vi "KeepScreenTrunOn.vi"(8 "error in (no error)":errorcluster) -> (0 "error out":errorcluster, 3 "PowerHandle":u32)   [LabVIEW 2020, in "Power Requests.lvlib"]
uses:
  Power Requests.lvlib
  Power Availabilty Requests/Type Defs/Power Request Type.ctl
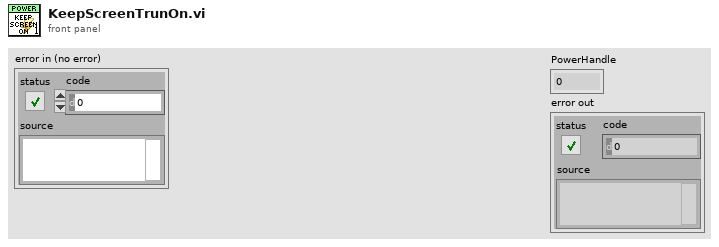
[diagram p1: front panel]
types:
  T1 = typedef "Power Requests.lvlib/Power Request Type.ctl" = enum32{"Power Request Display Required", "Power Request System Required", "Power Request Away Mode Required", "Power Request Execution Required"}
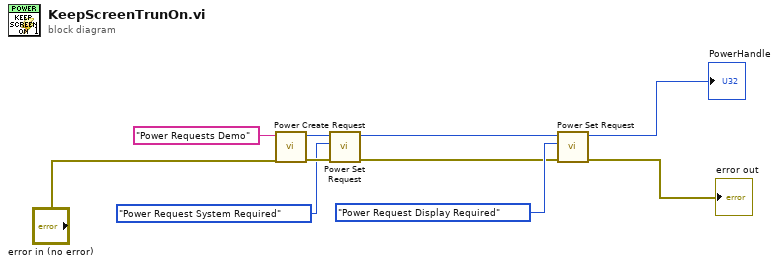
[diagram p0: block diagram]
diagram:
  n1 = call "Power Create Request.vi"("error in (no error)"="error in (no error)", "Simple Reason String"="Power Requests Demo") -> ("error out"=w10:errorcluster, "Handle"=w9:i64)  [unwired: 8 in]
  n2 = call "Power Set Request.vi"("error in (no error)"=w10, "Power Request Type"=Power_Request_Type."Power Request System Required", "Handle in"=w9) -> ("error out"=w5:errorcluster, "Handle out"=w4:u32)  [unwired: 6 in, 1 out]
  n3 = call "Power Set Request.vi"("error in (no error)"=w5, "Power Request Type"=Power_Request_Type."Power Request Display Required", "Handle in"=w4) -> ("error out"=→"error out":errorcluster, "Handle out"=→"PowerHandle":u32)  [unwired: 6 in, 1 out]
